vi "FIND DEVICE FOR USEING.vi"(9 "product type":string[](array[string]), 11 "DAQmx Device Name":tag) -> (2 "T button?":bool, 3 "DAQmx Device Name OUT":tag)   [LabVIEW 2011]
uses:
  C:/Program Files/National Instruments/LabVIEW 8.6/resource/objmgr/daqmx.rc
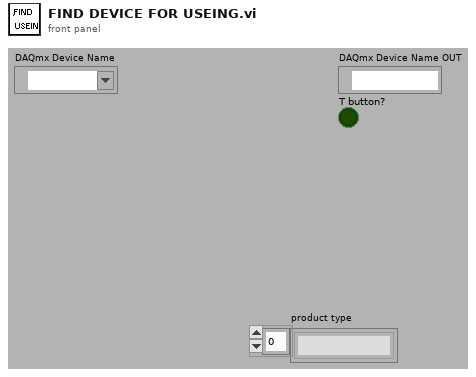
[diagram p1: front panel]
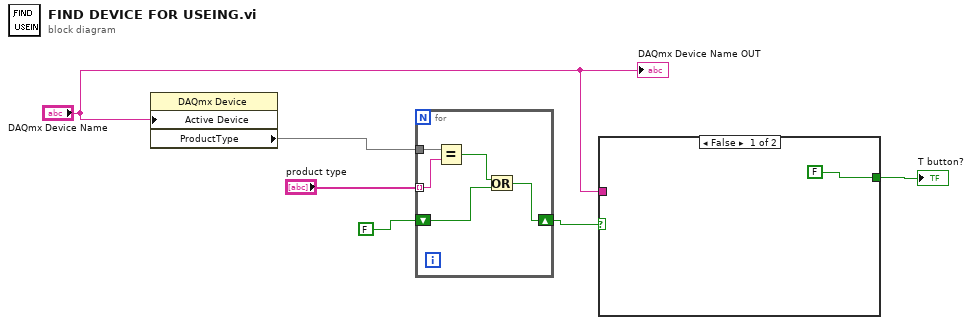
[diagram p0: block diagram]
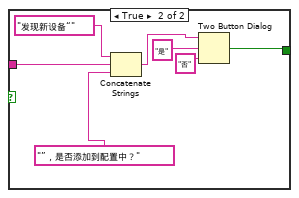
[diagram p2: hidden frame]
diagram:
  n1 = property class="DAQmx Device"("Active Device"="DAQmx Device Name") -> ("ProductType"=w6)  [unwired: 2 in, 2 out]
  n2 = for {
    tunnel: w6 -> [w11]
    tunnel: "product type" -> [w10] mode=indexing
    shift-right: [w7] -> w3
    shift-left: FALSE -> [w8]
    n3 = Equal?(x=w11, y=w10) -> (x = y?=w9:bool)
    n4 = Or(x=w9, y=w8) -> (x .or. y?=w7:bool)
  }
  n5 = case shown="False" w3 {
    tunnel: "DAQmx Device Name" -> [_ w18]
    tunnel: [FALSE w13] -> w1
    frame False {
    }
    frame True {
      n6 = Concatenate Strings("发现新设备“", w18, "”，是否添加到配置中？") -> (w16:string)
      n7 = Two Button Dialog(message=w16, 1:"否" ("F button name (\"Cancel\")"), 2:"是" ("T button name (\"OK\")")) -> (T button?=w13:bool)
    }
  }
  "T button?" <- w1
  "DAQmx Device Name OUT" <- "DAQmx Device Name"
